vi "区域判断.vi"(4 "压力数组":dbl[](array[numeric]), 5 "位移数组":dbl[](array[numeric]), 6 "区域最大压力":dbl, 7 "区域最小压力":dbl, 8 "区域最大位移":dbl, 9 "区域最小位移":dbl) -> (3 "区域监控合格":bool)   [LabVIEW 2011]
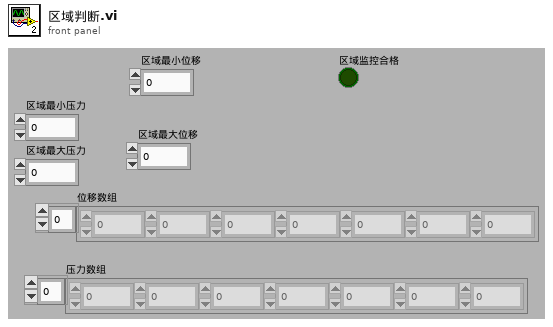
[diagram p1: front panel]
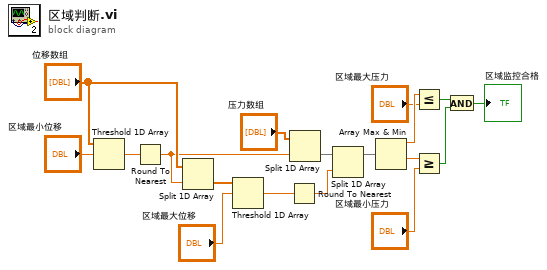
[diagram p0: block diagram]
diagram:
  n1 = Threshold 1D Array(2:"区域最小位移", 3:"位移数组") -> (0:w16:dbl)  [unwired: 1 in]
  n2 = Round To Nearest(number=w16) -> (nearest integer value=w11:dbl)
  n3 = Split 1D Array(array="位移数组", index=w11) -> (second subarray=w12:dbl[])  [unwired: 1 out]
  n4 = Threshold 1D Array(2:"区域最大位移", 3:w12) -> (0:w15:dbl)  [unwired: 1 in]
  n5 = Round To Nearest(number=w15) -> (nearest integer value=w9:dbl)
  n6 = Split 1D Array(array="压力数组", index=w11) -> (second subarray=w10:dbl[])  [unwired: 1 out]
  n7 = Split 1D Array(array=w10, index=w9) -> (first subarray=w8:dbl[])  [unwired: 1 out]
  n8 = Array Max & Min(array=w8) -> (max value=w7:dbl, min value=w5:dbl)  [unwired: 2 out]
  n9 = Less Or Equal?(x=w7, y="区域最大压力") -> (x <= y?=w3:bool)
  n10 = Greater Or Equal?(x=w5, y="区域最小压力") -> (x >= y?=w2:bool)
  n11 = And(x=w3, y=w2) -> (x .and. y?=→"区域监控合格":bool)
